vi "run_imagecollection.vi"(8 "error in (no error)":errorcluster, 11 "AnalysisRAPS in":refnum<class "AnalysisRAPS.lvclass">) -> (0 "error out":errorcluster, 3 "AnalysisRAPS out":refnum<class "AnalysisRAPS.lvclass">)   [LabVIEW 2010, in "AnalysisRAPS.lvclass"]
uses:
  AnalysisRAPS.lvclass
  common/classes/ImageCollection/ImageCollection/ImageCollection.lvclass
  common/classes/Image/Image/Image.lvclass
  AnalysisRAPS.lvclass/AnalysisRAPS.ctl
  saving_type.ctl
panel:
  in  "average":i32=1 min=1 step=1
  in  "button:stop":bool
  out "Image":T1(plugin-control)
  in  "Path":path
  out "Slide":u8(slide) scale=0.0..100.0
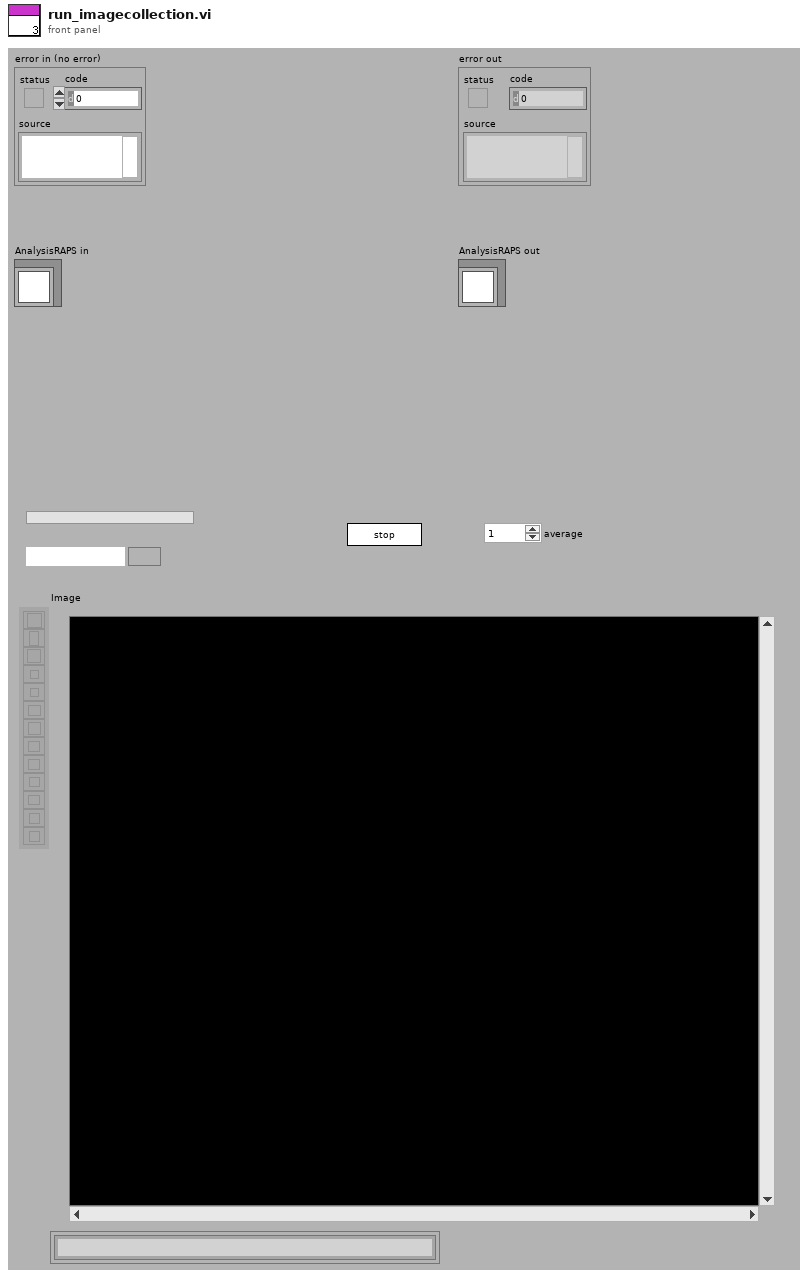
[diagram p1: front panel]
types:
  T1 = typedef "IMAQ Image.ctl" = refnum<image>
  T2 = typedef "AnalysisRAPS.lvclass/saving_type.ctl" = enum16{"raw", "average"}
  T3 = typedef "Image Type" = u32
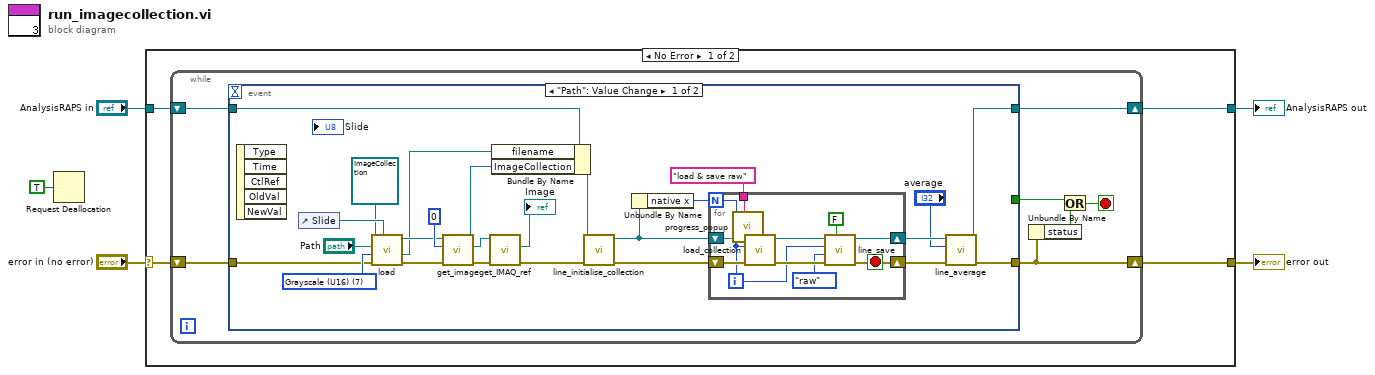
[diagram p0: block diagram]
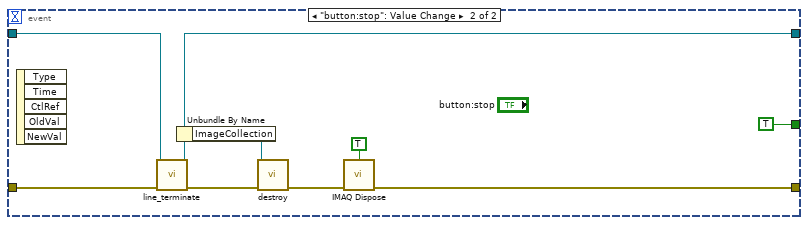
[diagram p2: hidden frame]
diagram:
  n1 = Request Deallocation(TRUE ("flag")) -> ()
  n2 = case shown="No Error" "error in (no error)" {
    selector: "error in (no error)" -> [w8 w63]
    tunnel: [w9 w63] -> w4
    tunnel: [w7 w62] -> w2
    tunnel: "AnalysisRAPS in" -> [w6 w62]
    frame No Error {
      n3 = while {
        shift-right: [w13] -> w9
        shift-left: w8 -> [w16]
        shift-right: [w15] -> w7
        shift-left: w6 -> [w14]
        stop <- w11 stop-if-true
        n4 = event shown="[0] \"Path\": Value Change" {
          selector: _ -> [_ _]
          dyn-events: _ -> [_ _]
          timeout: _ -> [_ _]
          tunnel: [w23 w54] -> w13
          tunnel: w16 -> [w30 w56]
          tunnel: [w25 w58] -> w15
          tunnel: w14 -> [w38 w59]
          tunnel: [_ TRUE] -> w10
          event "Path": Value Change {
            w39 = T3 7 items=["Grayscale (U8)", "Grayscale (I16)", "Grayscale (SGL)", "Complex (CSG)", "RGB (U32)", "HSL (U32)", "RGB (U64)", "Grayscale (U16)"] ("Image Type")
            n5 = event-data() -> ()  [unwired: 1 in, 5 out]
            n6 = control-ref of="Slide"() -> (w41:refnum<vi>)
            n7 = call "load.vi"("progress bar ref"=w41, "error in (no error)"=w30, "Image Type"=w39, "path in"="Path", "ImageCollection in"=refnum<class "ImageCollection.lvclass"> refnum) -> ("error out"=w36:errorcluster, "path out"=w28:path, "ImageCollection out"=w32:refnum<class "ImageCollection.lvclass">)  [unwired: 2 in, 2 out]
            n8 = call-dynamic "get_image.vi"("error in (no error)"=w36, "index"=0, "ImageCollection in"=w32) -> ("error out"=w35:errorcluster, "Image.lvclass"=w34:refnum<class "Image.lvclass">, "ImageCollection out"=w31:refnum<class "ImageCollection.lvclass">)  [unwired: 6 in]
            n9 = call-dynamic "get_IMAQ_ref.vi"("error in (no error)"=w35, "Image.lvclass in"=w34) -> ("error out"=w19:errorcluster, "Image"=→"Image":T1)  [unwired: 5 in, 3 out]
            n10 = Bundle By Name(cluster=w38, "filename"=w28, "ImageCollection"=w31) -> (w20:refnum<class "AnalysisRAPS.lvclass">)
            n11 = call-dynamic "line_initialise_collection.vi"("error in (no error)"=w19, "AnalysisRAPS in"=w20) -> ("error out"=w17:errorcluster, "AnalysisRAPS out"=w18:refnum<class "AnalysisRAPS.lvclass">)  [unwired: 8 in]
            n12 = Unbundle By Name(w18) -> ("native x"=w27:i32)
            n13 = for {
              N: w27 -> [w46]
              shift-right: [w49] -> w26
              shift-left: w18 -> [w52]
              shift-right: [w47] -> w24
              shift-left: w17 -> [w51]
              tunnel: "load & save raw" -> [w44]
              i -> [w45]
              stop <- w47 stop-if-true
              n14 = call "progress_popup.vi"("custom text"=w44, "current"=w45, "total"=w46) -> ()  [unwired: 9 in]
              n15 = call-dynamic "load_collection.vi"("error in (no error)"=w51, "index"=w45, "AnalysisRAPS in"=w52) -> ("error out"=w48:errorcluster, "AnalysisRAPS out"=w50:refnum<class "AnalysisRAPS.lvclass">)  [unwired: 7 in]
              n16 = call-dynamic "line_save.vi"("double? (F)"=FALSE, "error in (no error)"=w48, "save type"=saving_type."raw", "index"=w45, "AnalysisRAPS in"=w50) -> ("error out"=w47:errorcluster, "AnalysisRAPS out"=w49:refnum<class "AnalysisRAPS.lvclass">)  [unwired: 5 in]
            }
            n17 = call-dynamic "line_average.vi"("error in (no error)"=w24, "average"="average", "AnalysisRAPS in"=w26) -> ("error out"=w23:errorcluster, "AnalysisRAPS out"=w25:refnum<class "AnalysisRAPS.lvclass">)  [unwired: 7 in]
          }
          event "button:stop": Value Change {
            n18 = event-data() -> ()  [unwired: 1 in, 5 out]
            n19 = call-dynamic "line_terminate.vi"("error in (no error)"=w56, "AnalysisRAPS in"=w59) -> ("error out"=w57:errorcluster, "AnalysisRAPS out"=w58:refnum<class "AnalysisRAPS.lvclass">)  [unwired: 8 in]
            n20 = Unbundle By Name(w58) -> ("ImageCollection"=w60:refnum<class "ImageCollection.lvclass">)
            n21 = call-dynamic "destroy.vi"("error in (no error)"=w57, "ImageCollection in"=w60) -> ("error out"=w55:errorcluster)  [unwired: 8 in, 1 out]
            n22 = call "IMAQ Dispose"("All Images? (No)"=TRUE, "error in (no error)"=w55) -> ("error out"=w54:errorcluster)  [unwired: 4 in]
          }
        }
        n23 = Unbundle By Name(w13) -> ("status"=w12:bool)
        n24 = Or(x=w10, y=w12) -> (x .or. y?=w11:bool)
      }
    }
    frame Error {
    }
  }
  "error out" <- w4
  "AnalysisRAPS out" <- w2
